vi "niScope Configure Trigger Edge.vi"(0 "instrument handle":refnum<k15>, 1 "trigger slope":T3, 2 "trigger coupling":T2=1 items=["AC"=0, "DC"=1, "HF Reject"=3, "LF Reject"=4, "AC Plus HF Reject"=1001], 5 "trigger source":T1="0" caption="trigger source (Channel 0)", 7 "trigger level":dbl format="%.2f", 11 "error in":errorcluster, 12 "trigger holdoff":dbl format="%.4f", 13 "trigger delay":dbl format="%.4f") -> (4 "instrument handle out":refnum<k15>, 15 "error out":errorcluster)   [LabVIEW 2011]
doc: "Configures common properties for edge triggering."
uses:
  <instrlib>/niScope/Controls/niScope trigger slope.ctl
  <instrlib>/niScope/Controls/niScope trigger coupling.ctl
  <instrlib>/niScope/Controls/niScope trigger source.ctl
  niScope_32.dll
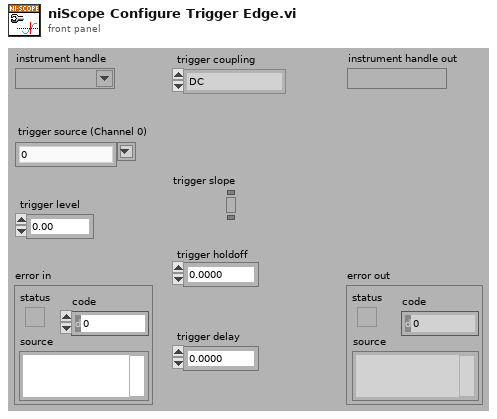
[diagram p1: front panel]
types:
  T1 = typedef "niScope trigger source.ctl" = string
  T2 = typedef "niScope trigger coupling.ctl" = u16
  T3 = typedef "niScope trigger slope.ctl" = i32
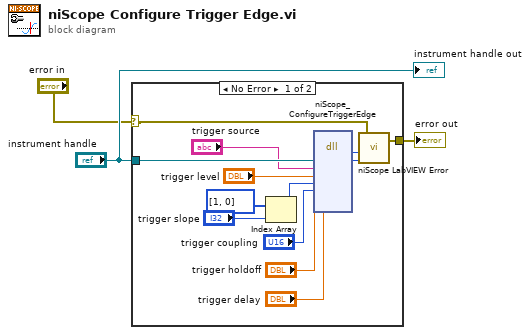
[diagram p0: block diagram]
diagram:
  n1 = case shown="No Error" "error in" {
    selector: "error in" -> [w5 w17]
    tunnel: [w13 w17] -> w3
    tunnel: "instrument handle" -> [w16 _]
    frame No Error {
      n2 = Index Array(array=i32[] [1, 0] ("trigger slope arr"), index="trigger slope") -> (element=w11:i32)
      n3 = dll-call lib="niScope_*.*" fn="niScope_ConfigureTriggerEdge"("instrument handle"=w16, "triggerSource"="trigger source", "level"="trigger level", "slope"=w11, "coupling"="trigger coupling", "holdoff"="trigger holdoff", "delay"="trigger delay") -> ("status"=w15:i32, "instrument handle"=w14:u32)  [unwired: 9 in, 2 out]
      n4 = call <instrlib>:"niScope LabVIEW Error.vi"("instrument handle"=w14, "niScope error code (0)"=w15, "error in (no error)"=w5) -> ("error out"=w13:errorcluster)  [unwired: 2 in]
    }
    frame Error {
    }
  }
  "error out" <- w3
  "instrument handle out" <- "instrument handle"
